vi "Creat new log or directory.vi"(8 "error in":errorcluster, 11 "Log":path=path "C:/Users/ANNIE/Documents/Logs/Channel Logs") -> (0 "error out":errorcluster, 3 "New Log":path)   [LabVIEW 2018]
uses:
  <userlib>/_OpenG.lib/file/file.llb/File Exists - Scalar__ogtk.vi
  <vilib>/regexp/Match Regular Expression.xnode
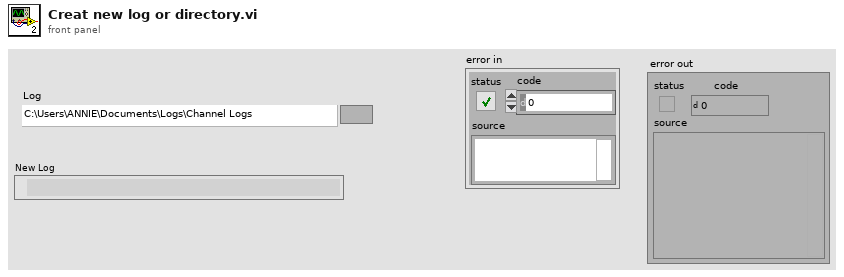
[diagram p1: front panel]
types:
  T1 = enum16{"open", "replace", "create", "open or create", "replace or create", "replace or create with confirmation"}
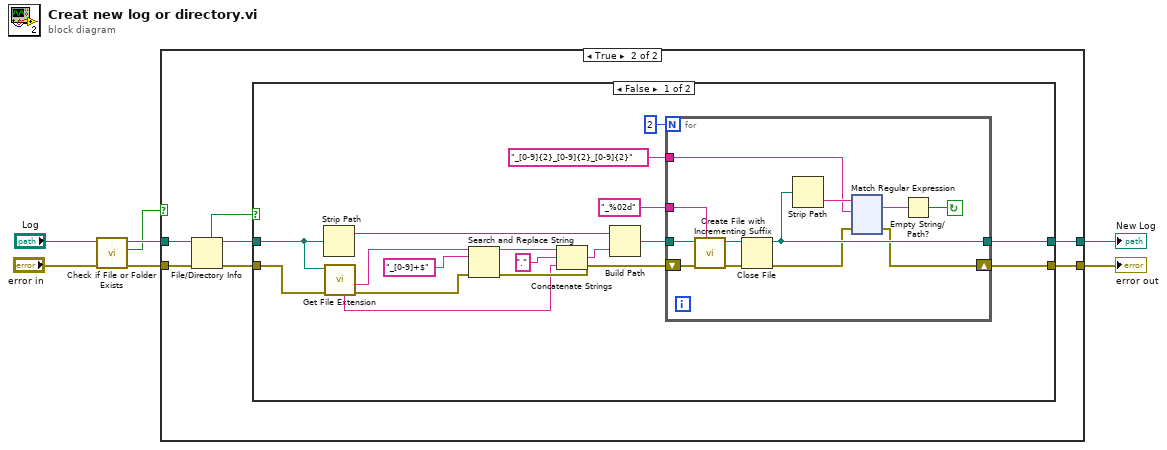
[diagram p0: block diagram]
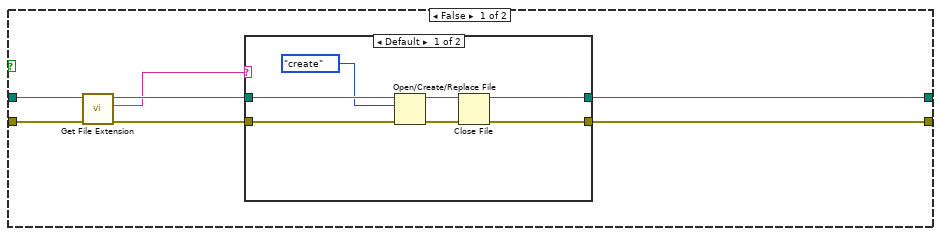
[diagram p2: hidden frame]
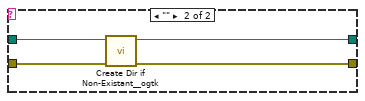
[diagram p3: hidden frame]
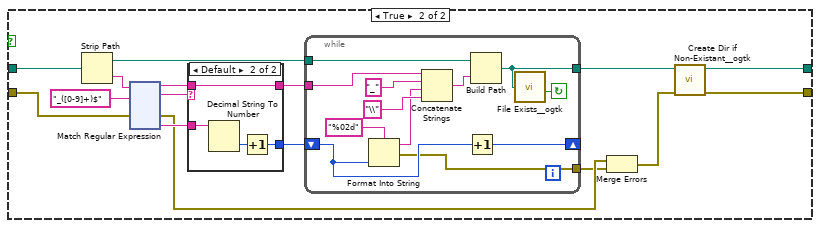
[diagram p4: hidden frame]
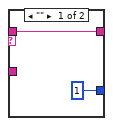
[diagram p5: hidden frame]
diagram:
  n1 = call <vilib>:"Check if File or Folder Exists.vi"("error in (no error)"="error in", "path"="Log") -> ("error out"=w2:errorcluster, "file or folder exists?"=w1:bool, "dup path"=w3:path)  [unwired: 7 in]
  n2 = case shown="True" w1 {
    tunnel: [w9 w32] -> w7
    tunnel: [w8 w31] -> w6
    tunnel: w3 -> [w13 w30]
    tunnel: w2 -> [w14 w29]
    frame False {
      n3 = call <vilib>:"Get File Extension.vi"("error in (no error)"=w14, "file"=w13) -> ("error out"=w10:errorcluster, "lowercase file extension"=w11:string, "dup file"=w12:path)  [unwired: 5 in, 2 out]
      n4 = case shown="Default" w11 {
        tunnel: w12 -> [w20 w25]
        tunnel: w10 -> [w21 w24]
        tunnel: [w16 w23] -> w9
        tunnel: [w15 w22] -> w8
        frame Default {
          n5 = Open/Create/Replace File(file path (use dialog)=w20, error in=w21, operation (0:open)=T1."create") -> (refnum out=w17:refnum<file>, error out=w18:errorcluster)  [unwired: 3 in, 1 out]
          n6 = Close File(refnum=w17, error in=w18) -> (path=w15:path, error out=w16:errorcluster)
        }
        frame "" {
          n7 = call <userlib>:"Create Dir if Non-Existant__ogtk.vi"("error in (no error)"=w24, "Directory Path"=w25) -> ("error out"=w23:errorcluster, "dup Directory Path"=w22:path)  [unwired: 7 in, 1 out]
        }
      }
    }
    frame True {
      n8 = File/Directory Info(path=w30, error in=w29) -> (path out=w27:path, directory=w26:bool, error out=w28:errorcluster)  [unwired: 4 out]
      n9 = case shown="False" w26 {
        tunnel: [w36 w189] -> w32
        tunnel: [w37 w186] -> w31
        tunnel: w27 -> [w45 w185]
        tunnel: w28 -> [w40 w179]
        frame False {
          n10 = Strip Path(path=w45) -> (stripped path=w49:path)  [unwired: 1 out]
          n11 = call <vilib>:"Get File Extension.vi"("error in (no error)"=w40, "file"=w45) -> ("error out"=w39:errorcluster, "filename without extension"=w44:string, "unmodified file extension"=w41:string)  [unwired: 5 in, 2 out]
          n12 = Search and Replace String(input string=w44, search string="_[0-9]+$" ("format string (\" (%d)\")"), error in=w39) -> (result string=w43:string, error out=w47:errorcluster)  [unwired: 5 in, 2 out]
          n13 = Concatenate Strings(w43, "." ("result string"), w41) -> (w42:string)
          n14 = Build Path(base path=w49, name or relative path=w42) -> (appended path=w48:path)
          n15 = for {
            N: 2 -> [_]
            tunnel: w48 -> [w61]
            tunnel: [w56] -> w37
            shift-right: [w52] -> w36
            shift-left: w47 -> [w60]
            tunnel: "_%02d" ("format string (\" (%d)\")") -> [w57]
            tunnel: "_[0-9]{2}_[0-9]{2}_[0-9]{2}" ("format string (\" (%d)\")") -> [w54]
            stop <- w50 continue-if-true
            n16 = call <vilib>:"Create File with Incrementing Suffix.vi"("format string (\" (%d)\")"=w57, "error in (no error)"=w60, "file path"=w61) -> ("error out"=w59:errorcluster, "refnum out"=w58:refnum<file>)  [unwired: 6 in, 1 out]
            n17 = Close File(refnum=w58, error in=w59) -> (path=w56:path, error out=w53:errorcluster)
            n18 = Strip Path(path=w56) -> (name=w55:string)  [unwired: 1 out]
            n19 = xnode "Match Regular Expression"("input string"=w55, "regular expression"=w54, "error in"=w53) -> ("whole match"=w51:string, "error out"=w52:errorcluster)  [unwired: 3 in, 3 out]
            n20 = Empty String/Path?(string/path=w51) -> (empty?=w50:bool)
          }
        }
        frame True {
          n21 = Strip Path(path=w185) -> (stripped path=w191:path, name=w188:string)
          n22 = xnode "Match Regular Expression"("input string"=w188, "regular expression"="_([0-9]+)$", "error in"=w179) -> ("before match"=w181:string, "whole match"=w184:string, "error out"=w178:errorcluster, "submatch 1"=w183:string)  [unwired: 3 in, 2 out]
          n23 = case shown="Default" w184 {
            tunnel: w183 -> [_ w208]
            tunnel: [1 w207] -> w182
            tunnel: [w204 w206] -> w180
            tunnel: w181 -> [w204 w206]
            frame "" {
            }
            frame Default {
              n24 = Decimal String To Number(string=w208) -> (number=w209:i32)  [unwired: 2 in, 1 out]
              n25 = Increment(x=w209) -> (x+1=w207:i32)
            }
          }
          n26 = while {
            tunnel: w180 -> [w198]
            tunnel: w191 -> [w201]
            tunnel: [w199] -> w190
            shift-right: [w196] -> _
            shift-left: w182 -> [w194]
            tunnel: [w193] -> w177
            stop <- w197 continue-if-true
            n27 = Format Into String(format string="%02d" ("regular expression"), w194) -> (resulting string=w195:string, error out=w193:errorcluster)  [unwired: 2 in]
            n28 = Concatenate Strings(w198, "_" ("regular expression"), w195, "\\" ("regular expression")) -> (w202:string)
            n29 = Increment(x=w194) -> (x+1=w196:i32)
            n30 = Build Path(base path=w201, name or relative path=w202) -> (appended path=w199:path)
            n31 = call-poly <userlib>:"File Exists__ogtk.vi"("file path"=w199) -> ("exists"=w197:bool)  [unwired: 6 in, 1 out]
          }
          n32 = Merge Errors(w178, w177) -> (w176:errorcluster)
          n33 = call <userlib>:"Create Dir if Non-Existant__ogtk.vi"("error in (no error)"=w176, "Directory Path"=w190) -> ("error out"=w189:errorcluster, "dup Directory Path"=w186:path)  [unwired: 7 in, 1 out]
        }
      }
    }
  }
  "error out" <- w7
  "New Log" <- w6
